vi "add event.vi"(0 "Mode":bool, 1 "TBM 5":string[][](array[string]), 2 "Subtask":u16, 3 "Combo Box":T2="Cancelled", 5 "Additional info":string, 6 "List of robots":T1="UGV1-Raptor", 8 "Subtask registered event in":string[][](array[string])) -> (14 "Subtask registered event out":T2[][](array[typedef]), 15 "TBM 4":string[][](array[string]))   [LabVIEW 2015, in "Biblioteka moduł map v3.lvlib" / "task erl.lvlib"]
uses:
  task erl.lvlib
  Status task.ctl
  List of robots.ctl
  Zmienne/Lokalizacja GPS/latitude.vi
  Zmienne/Lokalizacja GPS/longitude.vi
  Zmienne/Lokalizacja GPS/longitude Quadron.vi
  Zmienne/Lokalizacja GPS/latitude Quadron.vi
  Zmienne/Lokalizacja GPS/Latitude dron 1.vi
  Zmienne/Lokalizacja GPS/Longitude dron 1.vi
  Zmienne/Lokalizacja GPS/Longitude dron 2.vi
  Zmienne/Lokalizacja GPS/Latitude dron 2.vi
  Zmienne/Lokalizacja GPS/Latitude Sparus.vi
  Zmienne/Lokalizacja GPS/Longitude Sparus.vi
  KML/KML.lvlib
  Zmienne/Lokalizacja GPS/Lokalizacja GPS.lvlib
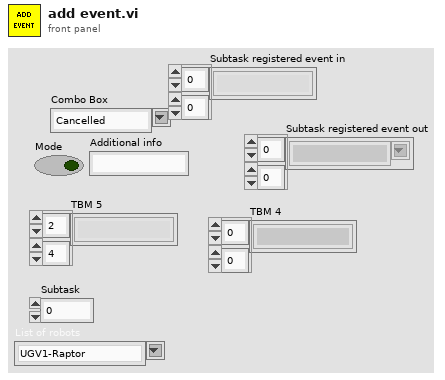
[diagram p1: front panel]
types:
  T1 = typedef "Biblioteka moduł map v3.lvlib/task erl.lvlib/List of robots.ctl" = string
  T2 = typedef "Biblioteka moduł map v3.lvlib/task erl.lvlib/Status task.ctl" = string
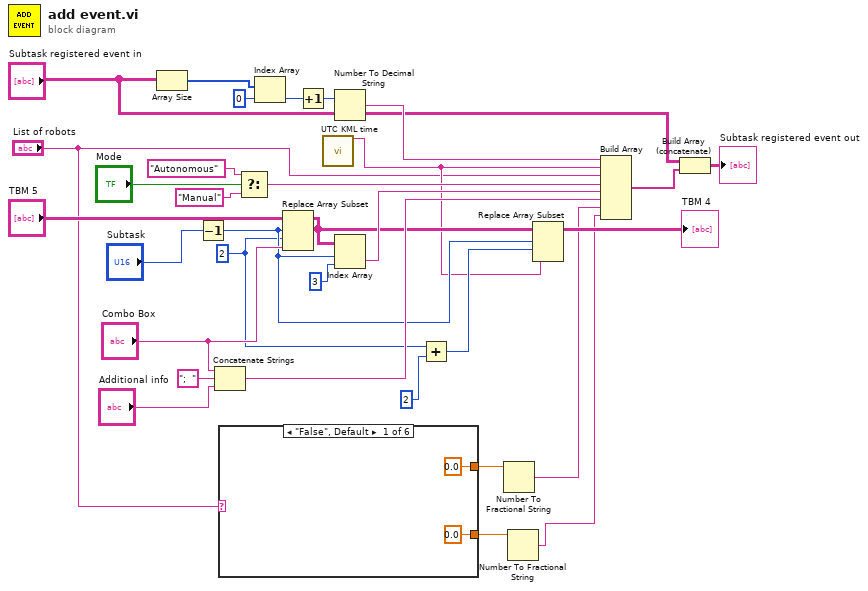
[diagram p0: block diagram]
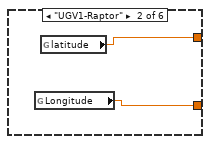
[diagram p2: hidden frame]
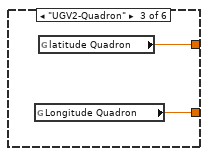
[diagram p3: hidden frame]
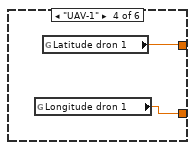
[diagram p4: hidden frame]
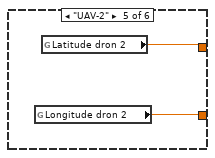
[diagram p5: hidden frame]
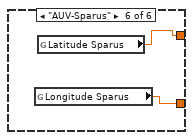
[diagram p6: hidden frame]
diagram:
  w10 = 2 ("disabled index (col)")
  n1 = Array Size(array="Subtask registered event in") -> (size(s)=w25:i32[])
  n2 = Decrement(x="Subtask") -> (x-1=w11:u16)
  n3 = Concatenate Strings("Combo Box", ";  " ("string"), "Additional info") -> (w15:string)
  n4 = case shown="\"False\", Default" "List of robots" {
    tunnel: [0.0 ("Latitude Sparus") w36 w38 w40 w42 w44] -> w2
    tunnel: [0.0 ("Longitude Sparus") w35 w37 w39 w41 w43] -> w1
    frame "False", Default {
    }
    frame "UGV1-Raptor" {
      n5 = global read "longitude.vi" "Longitude"() -> (w35:dbl)
      n6 = global read "latitude.vi" "latitude"() -> (w36:dbl)
    }
    frame "UGV2-Quadron" {
      n7 = global read "longitude Quadron.vi" "Longitude Quadron"() -> (w37:dbl)
      n8 = global read "latitude Quadron.vi" "latitude Quadron"() -> (w38:dbl)
    }
    frame "UAV-1" {
      n9 = global read "Longitude dron 1.vi" "Longitude dron 1"() -> (w39:dbl)
      n10 = global read "Latitude dron 1.vi" "Latitude dron 1"() -> (w40:dbl)
    }
    frame "UAV-2" {
      n11 = global read "Longitude dron 2.vi" "Longitude dron 2"() -> (w41:dbl)
      n12 = global read "Latitude dron 2.vi" "Latitude dron 2"() -> (w42:dbl)
    }
    frame "AUV-Sparus" {
      n13 = global read "Longitude Sparus.vi" "Longitude Sparus"() -> (w43:dbl)
      n14 = global read "Latitude Sparus.vi" "Latitude Sparus"() -> (w44:dbl)
    }
  }
  n15 = Select(t="Autonomous", s="Mode", f="Manual") -> (s? t:f=w29:string)
  n16 = Index Array(array=w25, index=0) -> (element=w23:i32)
  n17 = Replace Array Subset(array="TBM 5", new element="Combo Box", index (row)=w11, index (col)=w10) -> (w13:string[][])
  n18 = Increment(x=w23) -> (x+1=w22:i32)
  n19 = call "UTC KML time.vi"() -> ("String"=w7:string)  [unwired: 19 in]
  n20 = Number To Decimal String(number=w22) -> (decimal integer string=w21:string)  [unwired: 1 in]
  n21 = Index Array(array=w13, index (row)=w11, index (col)=3 ("disabled index (col)")) -> (element=w27:string)
  n22 = Add(x=w10, y=2) -> (x+y=w8:i32)
  n23 = Number To Fractional String(number=w2) -> (F-format string=w5:string)  [unwired: 3 in]
  n24 = Number To Fractional String(number=w1) -> (F-format string=w4:string)  [unwired: 3 in]
  n25 = Replace Array Subset(array=w13, new element=w7, index (row)=w11, index (col)=w8) -> (→"TBM 4":string[][])
  n26 = Build Array(w21, w7, "List of robots", w29, w27, w15, w5, w4) -> (w6:T1[])
  n27 = Build Array (concatenate)("Subtask registered event in", w6) -> (→"Subtask registered event out":T1[][])
